vi "Set Enabled Cameras.vi"(8 "error in (no error)":errorcluster, 10 "Cameras Enabled":bool[](array[boolean]), 11 "Application in":refnum<class "Application.lvclass">) -> (0 "error out":errorcluster, 3 "Application out":refnum<class "Application.lvclass">)   [LabVIEW 2018, in "Application.lvlib" / "Application.lvclass"]
uses:
  Application.lvclass
  Application.lvclass/Application.ctl
  Hardware/Hamamatsu Camera Messages/Set Enabled Cameras Msg/Set Enabled Cameras Msg.lvclass/Set Enabled Cameras Msg.ctl
  <vilib>/ActorFramework/Message Enqueuer/Message Enqueuer.lvclass/Message Enqueuer.ctl
  <vilib>/ActorFramework/Message Enqueuer/Enqueue.vi
  Hardware/Hamamatsu Camera Messages/Set Enabled Cameras Msg/Set Enabled Cameras Msg.lvclass
  C:/Program Files/National Instruments/LabVIEW 2018/vi.lib/ActorFramework/Message/Message.lvclass
  <vilib>/ActorFramework/Message Priority Queue/Priority Enqueue.vi
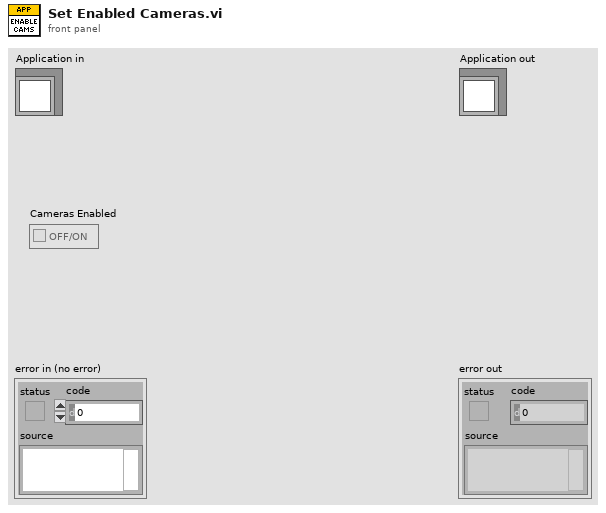
[diagram p1: front panel]
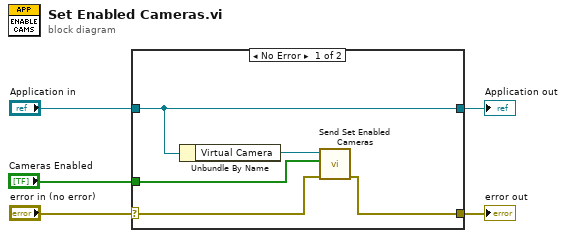
[diagram p0: block diagram]
diagram:
  n1 = case shown="No Error" "error in (no error)" {
    selector: "error in (no error)" -> [w8 w12]
    tunnel: [w7 w12] -> w4
    tunnel: [w10 w11] -> w2
    tunnel: "Application in" -> [w10 w11]
    tunnel: "Cameras Enabled" -> [w6 _]
    frame No Error {
      n2 = Unbundle By Name(w10) -> ("Virtual Camera"=w9:refnum<class "Message Enqueuer.lvclass">)
      n3 = call "Send Set Enabled Cameras.vi"("error in (no error)"=w8, "Cameras Enabled"=w6, "Message Enqueuer"=w9) -> ("error out"=w7:errorcluster)  [unwired: 7 in, 1 out]
    }
    frame Error {
    }
  }
  "error out" <- w4
  "Application out" <- w2
